vi "Configure Overcurrent Protection.vi"(6 "Delay Time (0.05 sec)":dbl=0.05, 7 "Enable Current Protection (T: Enable)":bool=TRUE, 8 "error in (no error)":errorcluster, 9 "Timer Start Moment (0: End Of Setting Change)":i32(ring) items=["End Of Setting Change", "Transition Into Constant Current Mode"], 10 "Channel (1)":string="1", 11 "VISA resource name":refnum<visa-resource-name>) -> (0 "error out":errorcluster, 3 "VISA resource name out":refnum<visa-resource-name>)   [LabVIEW 2020, in "Keysight E36300 Series.lvlib"]
doc: "Configures overcurrent protection."
uses:
  Keysight E36300 Series.lvlib
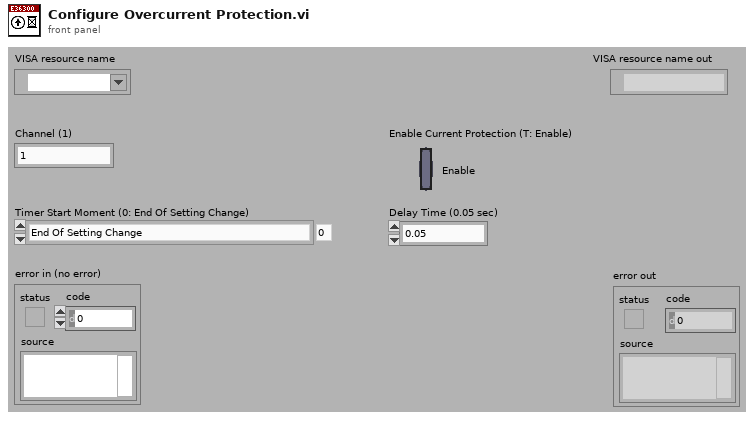
[diagram p1: front panel]
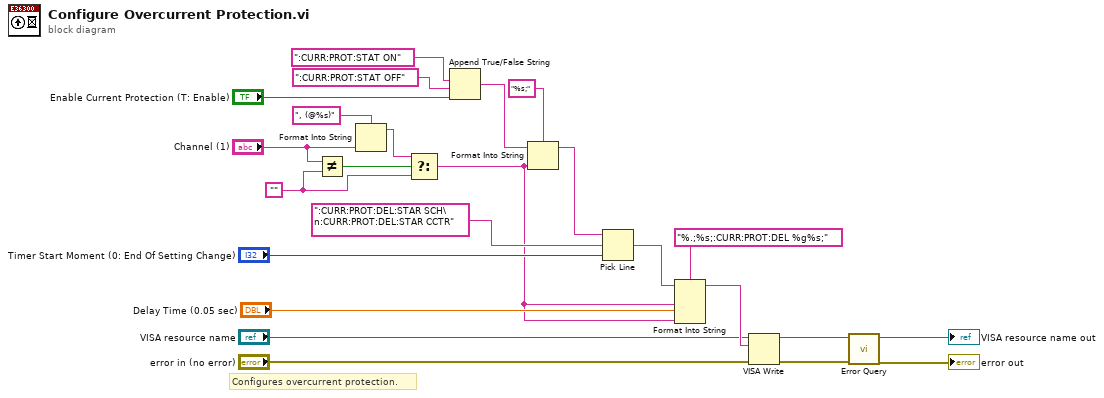
[diagram p0: block diagram]
diagram:
  w2 = ""
  # "Configures overcurrent protection."
  n1 = Not Equal?(x="Channel (1)", y=w2) -> (x != y?=w5:bool)
  n2 = Format Into String(format string=", (@%s)", "Channel (1)") -> (resulting string=w6:string)  [unwired: 2 in, 1 out]
  n3 = Select(t=w6, s=w5, f=w2) -> (s? t:f=w3:string)
  n4 = Append True/False String(1:"Enable Current Protection (T: Enable)", 2:":CURR:PROT:STAT OFF", 3:":CURR:PROT:STAT ON") -> (0:w10:string)  [unwired: 1 in]
  n5 = Format Into String(format string="%s;", initial string=w10, w3) -> (resulting string=w9:string)  [unwired: 1 in, 1 out]
  n6 = Pick Line(string ("")=w9, multi-line string=":CURR:PROT:DEL:STAR SCH\n:CURR:PROT:DEL:STAR CCTR", line index="Timer Start Moment (0: End Of Setting Change)") -> (output string=w19:string)
  n7 = Format Into String(format string="%.;%s;:CURR:PROT:DEL %g%s;", initial string=w19, w3, "Delay Time (0.05 sec)", w3) -> (resulting string=w17:string)  [unwired: 1 in, 1 out]
  n8 = VISA Write(VISA resource name="VISA resource name", write buffer=w17, error in (no error)="error in (no error)") -> (VISA resource name out=w14:refnum<visa-resource-name>, error out=w13:errorcluster)  [unwired: 1 out]
  n9 = call "Error Query.vi"("error in (no error)"=w13, "VISA resource name"=w14) -> ("error out"=→"error out":errorcluster, "VISA resource name out"=→"VISA resource name out":refnum<visa-resource-name>)  [unwired: 6 in, 2 out]
